vi "调整内边框位置和大小.vi"(8 "错误输入":errorcluster caption="错误输入（无错误）", 10 "窗口边界输入":T1 caption="窗口边界输出", 11 "引用":refnum<vi>) -> (0 "错误输出":errorcluster, 2 "窗口边界输出":T1 caption="窗口边界输入", 3 "引用输出":refnum<vi>)   [LabVIEW 8.6, in "窗口操作.lvlib"]
uses:
  <vilib>/Utility/miscctls.llb/LVRectTypeDef.ctl
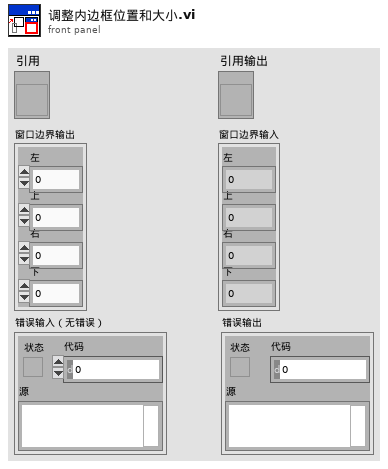
[diagram p1: front panel]
types:
  T1 = typedef "LVRectTypeDef.ctl" = cluster{"Left":i16, "Top":i16, "Right":i16, "Bottom":i16}
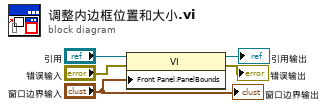
[diagram p0: block diagram]
diagram:
  n1 = property on="属性节点" class="VI"(reference="引用", error in="错误输入", "Front Panel.PanelBounds"="窗口边界输入") -> (reference out=→"引用输出":refnum<vi>, error out=→"错误输出":errorcluster)
  "窗口边界输出" <- "窗口边界输入"
